vi "Release Request.vi"(11 "INewConnectionCallback in":refnum<class "INewConnectionCallback.lvclass">) -> ()   [LabVIEW 2019, in "ConnectionFactorySession.lvlib" / "INewConnectionCallback.lvclass"]
uses:
  <vilib>/gpm_packages/@cs/Network-interface/Source/Connection Factory Session/INewConnectionCallback/INewConnectionCallback.lvclass
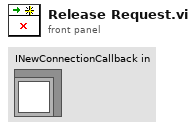
[diagram p1: front panel]
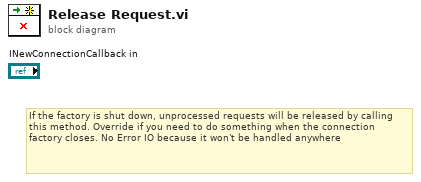
[diagram p0: block diagram]
diagram:
  # "If the factory is shut down, unprocessed requests will be released by calling this method. Override if you need to do something when the connection factory closes. No Error IO because it won't be handled anywhere"
